vi "generate name.vi"(10 "rest (T) active (F)":bool, 11 "Patient Name":string) -> (3 "appended path":path)   [LabVIEW 2014]
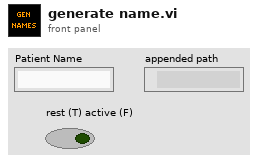
[diagram p1: front panel]
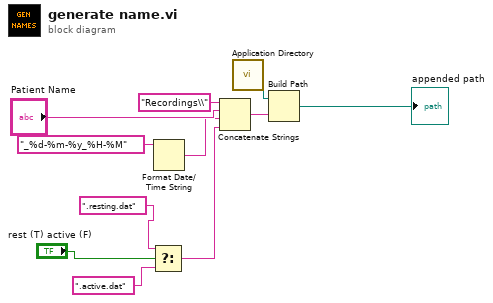
[diagram p0: block diagram]
diagram:
  n1 = Select(t=".resting.dat" ("string"), s="rest (T) active (F)", f=".active.dat" ("string")) -> (s? t:f=w2:string)
  n2 = Format Date/Time String(time format string (%c)="_%d-%m-%y_%H-%M") -> (date/time string=w6:string)  [unwired: 2 in]
  n3 = Concatenate Strings("Recordings\\" ("string"), "Patient Name", w6, w2) -> (w9:string)
  n4 = call <vilib>:"Application Directory.vi"() -> ("Application Directory"=w10:path)
  n5 = Build Path(base path=w10, name or relative path=w9) -> (appended path=→"appended path":path)
